vi "Measurement Logic.vi"(8 "error in":errorcluster, 9 "measurement configuration":T3={"double array in"=[3.4, 5.6], "double in"=1.2, "U32 array in"=[32, 33], "U32 in"=32, "U64 array in"=[64, 65], "U64 in"=64, "I32 array in"=[-32, -33], "I32 in"=-32, "I64 array in"=[-64, -65], "I64 in"=-64, "bool in"=TRUE, "string in"="Lorem ipsum dolor sit", "u32 color ring in"=1, "u32 animal enum in"=enum."Gopher"} {"u32 color ring in" items=["Red", "Green", "Blue"]}, 10 "measure call context in":refnum<class "Measure Call Context.lvclass">) -> (0 "error out":errorcluster, 1 "measurement results":T1={"xy data out"={"x_data"=[], "y_data"=[]}, "double array out"=[0.0], "double out"=0.0, "U32 array out"=[0], "U32 out"=0, "U64 array out"=[0], "U64 out"=0, "I32 array out"=[0], "I32 out"=0, "I64 array out"=[0], "I64 out"=0, "bool out"=FALSE, "string out"="Empty", "u32 color ring out"=0, "u32 animal enum out"=enum."Rabbit"} {"u32 color ring out" items=["Red", "Green", "Blue"]}, 2 "measure call context out":refnum<class "Measure Call Context.lvclass">)   [LabVIEW 2025, in "Automotive Ethernet Frame Generator.lvclass"]
doc: "Contains the core logic for executing the measurement."
uses:
  Automotive Ethernet Frame Generator.lvclass
  <vilib>/Plug-In SDKs/Measurements/Measure Call Context/Measure Call Context.lvclass
  Measurement Configuration.ctl
  Measurement Results.ctl
  <vilib>/gRPC/Generated APIs/ni/protobuf/types/RPC Messages/ni_protobuf_types_DoubleXYData.ctl
  <extravilib>/ChannelInstances/Event Messenger-bool/Instantiate.vi
  Automotive Ethernet Frame Generator.lvclass/Automotive Ethernet Frame Generator.ctl
  <vilib>/gRPC/Generated APIs/ni/protobuf/types/ni.protobuf.types.lvlib
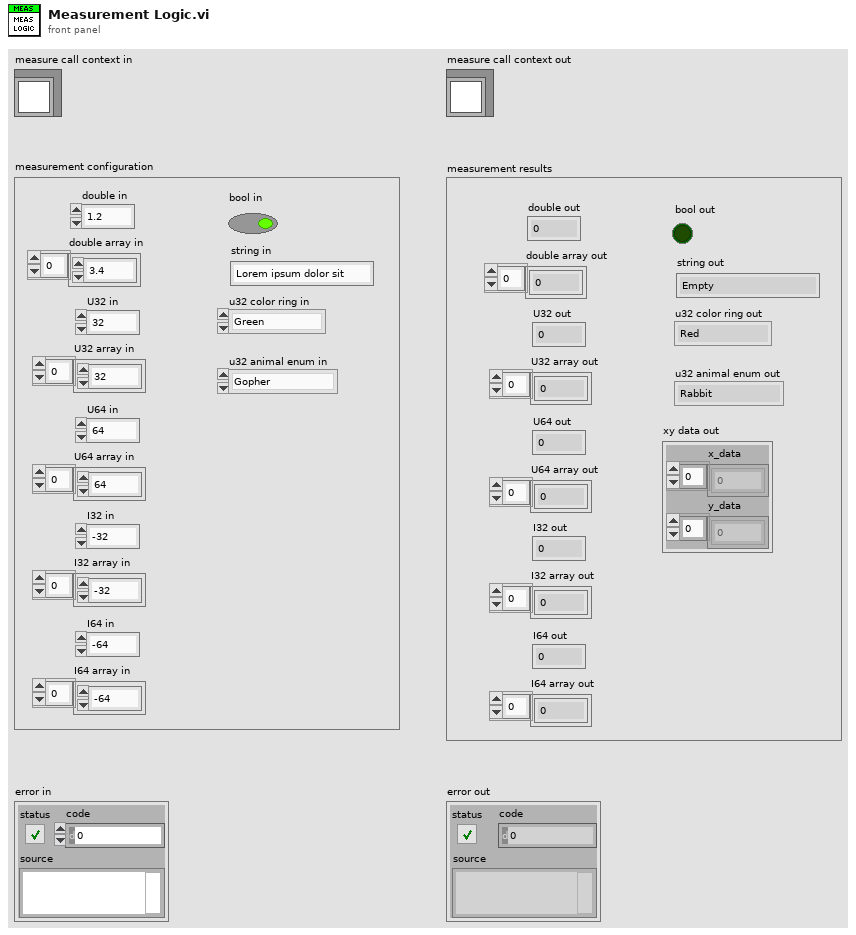
[diagram p1: front panel]
types:
  T1 = typedef "Automotive Ethernet Frame Generator.lvclass/Measurement Results.ctl" = cluster{"xy data out":T2, "double array out":dbl[], "double out":dbl, "U32 array out":u32[], "U32 out":u32, "U64 array out":u64[], "U64 out":u64, "I32 array out":i32[], "I32 out":i32, "I64 array out":i64[], "I64 out":i64, "bool out":bool, "string out":string, "u32 color ring out":u32, "u32 animal enum out":enum32{"Rabbit", "Gopher", "Badger"}}
  T2 = typedef "ni.protobuf.types.lvlib/ni_protobuf_types_DoubleXYData.ctl" = cluster{"x_data":dbl[], "y_data":dbl[]}
  T3 = typedef "Automotive Ethernet Frame Generator.lvclass/Measurement Configuration.ctl" = cluster{"double array in":dbl[], "double in":dbl, "U32 array in":u32[], "U32 in":u32, "U64 array in":u64[], "U64 in":u64, "I32 array in":i32[], "I32 in":i32, "I64 array in":i64[], "I64 in":i64, "bool in":bool, "string in":string, "u32 color ring in":u32, "u32 animal enum in":enum32{"Rabbit", "Gopher", "Badger"}}
  T4 = typedef "Event Messenger-bool.lvlib/))Channel.ctl" = refnum<queue>
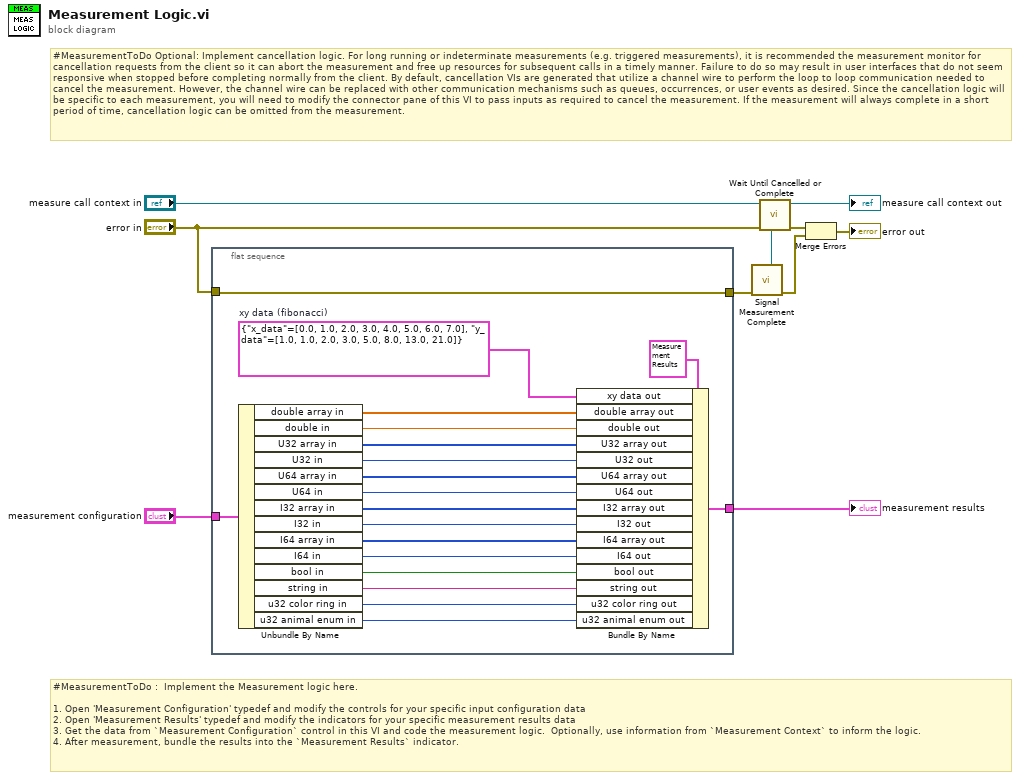
[diagram p0: block diagram]
diagram:
  # "#MeasurementToDo Optional: Implement cancellation logic. For long running or indeterminate measurements (e.g. triggered measurements), it is recommended the measurement monitor for cancellation requests from the client so it can abort the measurement and free up resources for subsequent calls in a timely manner. Failure to do so may result in user interfaces that do not seem responsive when stopped before completing normally from the client. By default, cancellation VIs are generated that utilize a channel wire to perform the loop to loop communication needed to cancel the measurement. However, the channel wire can be replaced with other communication mechanisms such as queues, occurrences, or user events as desired. Since the cancellation logic will be specific to each measurement, you will need to modify the connector pane of this VI to pass inputs as required to cancel the measurement. If the measurement will always complete in a short period of time, cancellation logic can be omitted from the measurement."
  # "#MeasurementToDo :  Implement the Measurement logic here.\n\n1. Open 'Measurement Configuration' typedef and modify the controls for your specific input configuration data\n2. Open 'Measurement Results' typedef and modify the indicators for your specific measurement results data\n3. Get the data from `Measurement Configuration` control in this VI and code the measurement logic.  Optionally, use information from `Measurement Context` to inform the logic.\n4. After measurement, bundle the results into the `Measurement Results` indicator."
  n1 = flat-sequence {
    tunnel: "measurement configuration" -> [w13]
    tunnel: [w12] -> w9
    tunnel: "error in" -> [w11]
    tunnel: [w11] -> w5
    frame #0 {
      w14 = T2 {"x_data"=[0.0, 1.0, 2.0, 3.0, 4.0, 5.0, 6.0, 7.0], "y_data"=[1.0, 1.0, 2.0, 3.0, 5.0, 8.0, 13.0, 21.0]}  # xy data (fibonacci)
      n2 = Unbundle By Name(w13) -> ("double array in"=w28:dbl[], "double in"=w27:dbl, "U32 array in"=w26:u32[], "U32 in"=w25:u32, "U64 array in"=w24:u64[], "U64 in"=w23:u64, "I32 array in"=w22:i32[], "I32 in"=w21:i32, "I64 array in"=w20:i64[], "I64 in"=w19:i64, "bool in"=w18:bool, "string in"=w17:string, "u32 color ring in"=w16:u32, "u32 animal enum in"=w15:enum32{"Rabbit", "Gopher", "Badger"})
      n3 = Bundle By Name(cluster=T1 {"xy data out"={"x_data"=[], "y_data"=[]}, "double array out"=[], "double out"=0.0, "U32 array out"=[0], "U32 out"=0, "U64 array out"=[0], "U64 out"=0, "I32 array out"=[0], "I32 out"=0, "I64 array out"=[0], "I64 out"=0, "bool out"=FALSE, "string out"="Empty", "u32 color ring out"=0, "u32 animal enum out"=enum."Rabbit"} ("Measurement Results"), "xy data out"=w14, "double array out"=w28, "double out"=w27, "U32 array out"=w26, "U32 out"=w25, "U64 array out"=w24, "U64 out"=w23, "I32 array out"=w22, "I32 out"=w21, "I64 array out"=w20, "I64 out"=w19, "bool out"=w18, "string out"=w17, "u32 color ring out"=w16, "u32 animal enum out"=w15) -> (w12:T1)
    }
  }
  n4 = call "Signal Measurement Complete.vi"("error in (no error)"=w5) -> ("error out"=w3:errorcluster, "done channel"=w4:T4)  [unwired: 9 in]
  n5 = call "Wait Until Cancelled or Complete.vi"("done channel"=w4, "error in (no error)"="error in", "measure call context in"="measure call context in") -> ("error out"=w2:errorcluster, "measure call context out"=→"measure call context out":refnum<class "Measure Call Context.lvclass">)  [unwired: 7 in]
  n6 = Merge Errors(w2, w3) -> (→"error out":errorcluster)
  "measurement results" <- w9
